vi "Untitled 3.vi"() -> ()   [LabVIEW 2013]
panel:
  in  "String":string
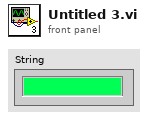
[diagram p1: front panel]
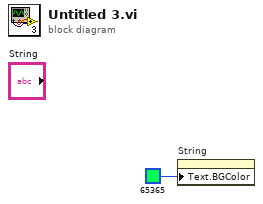
[diagram p0: block diagram]
diagram:
  n1 = property on="String" class="Str"("Text.BGColor"=u32 65365) -> ()  [unwired: 2 in, 2 out]
